vi "spectrometer-config.vi"(0 "Spectrograph Input Cluster":T3={"Slit Width (µm)"=50.0, "Diffraction Grating"=3, "Central Wavelength (nm)"=1000.0, "Filter"=4, "Shutter"=0} {"Shutter" items=["Close", "Open"]; "Slit Width (µm)" min=10.0 max=2500.0 step=0.1 format="%.1f"; "Diffraction Grating" items=["500 nm blaze"=1, "800 nm blaze"=2, "1250 nm blaze"=3]; "Filter" items=["Empty"=5, "Longpass 900 nm"=4, "Longpass 715 nm"=3, "Longpass 475 nm"=2, "Longpass 320 nm"=1]; "Central Wavelength (nm)" min=200.0 max=2000.0 step=0.1 format="%.1f"}, 2 "Initialization Successful?":bool, 3 "Spectrograph Reset Cluster":T1) -> (4 "Reset Control Cluster":T1, 5 "Spectrograph Output Cluster":T3={"Slit Width (µm)"=50.0, "Diffraction Grating"=3, "Central Wavelength (nm)"=1000.0, "Filter"=4, "Shutter"=0} {"Shutter" items=["Close", "Open"]; "Slit Width (µm)" min=10.0 max=2500.0 step=0.1 format="%.1f"; "Diffraction Grating" items=["500 nm blaze"=1, "800 nm blaze"=2, "1250 nm blaze"=3]; "Filter" items=["Empty"=5, "Longpass 900 nm"=4, "Longpass 715 nm"=3, "Longpass 475 nm"=2, "Longpass 320 nm"=1]; "Central Wavelength (nm)" min=200.0 max=2000.0 step=0.1 format="%.1f"}, 6 "Configuration Successful?":bool, 7 "Output Control Cluster":T2)   [LabVIEW 2015]
uses:
  <userlib>/Shamrock.llb/shamrock_autoSlit_typedef.ctl
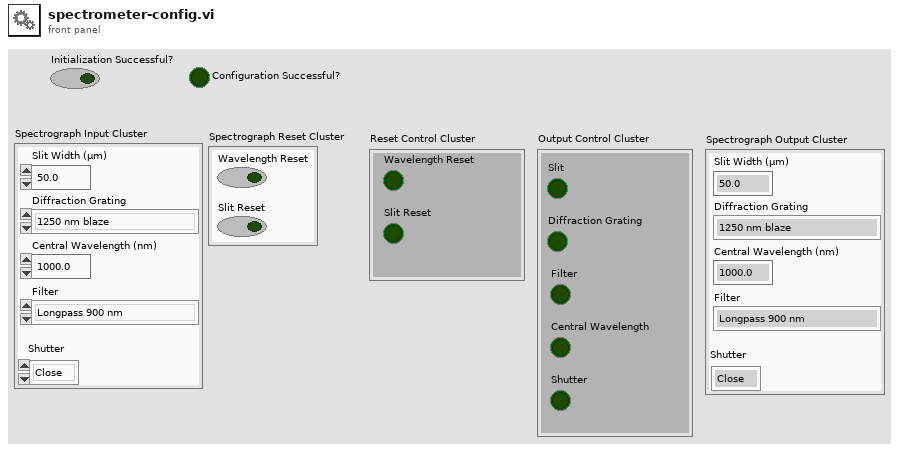
[diagram p1: front panel]
types:
  T1 = cluster{"Wavelength Reset":bool, "Slit Reset":bool}
  T2 = cluster{"Slit":bool, "Diffraction Grating":bool, "Filter":bool, "Central Wavelength":bool, "Shutter":bool}
  T3 = cluster{"Slit Width (µm)":dbl, "Diffraction Grating":u16, "Central Wavelength (nm)":dbl, "Filter":u16, "Shutter":u16}
  T4 = typedef "shamrock_autoSlit_typedef.ctl" = enum32{"Reserved (0)", "INPUT SIDE", "INPUT DIRECT", "OUTPUT SIDE", "OUTPUT DIRECT"}
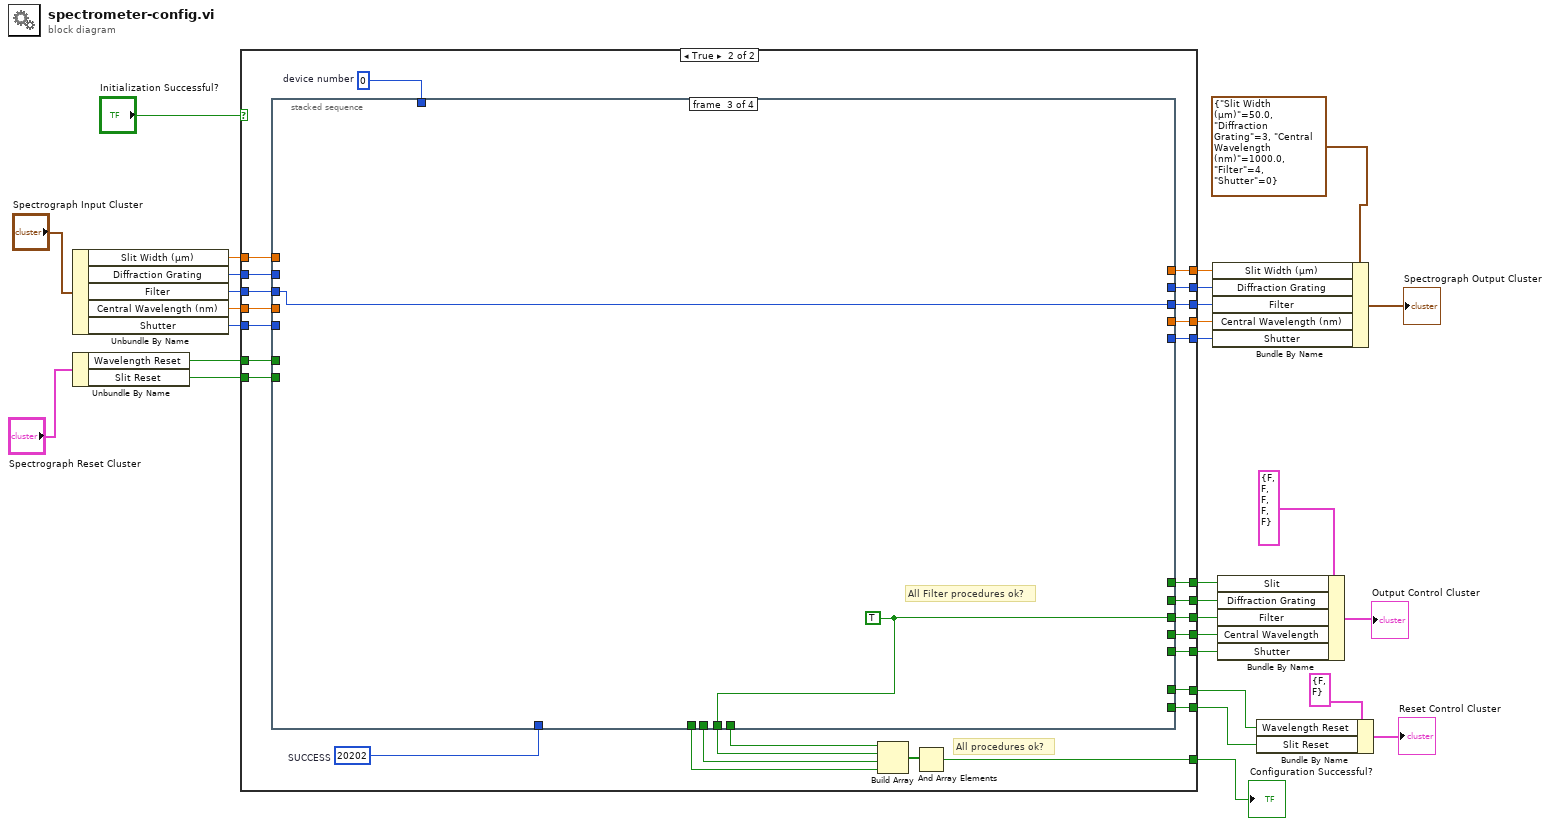
[diagram p0: block diagram]
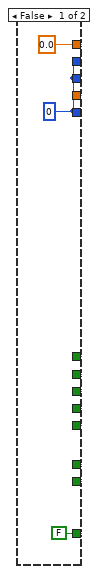
[diagram p2: hidden frame]
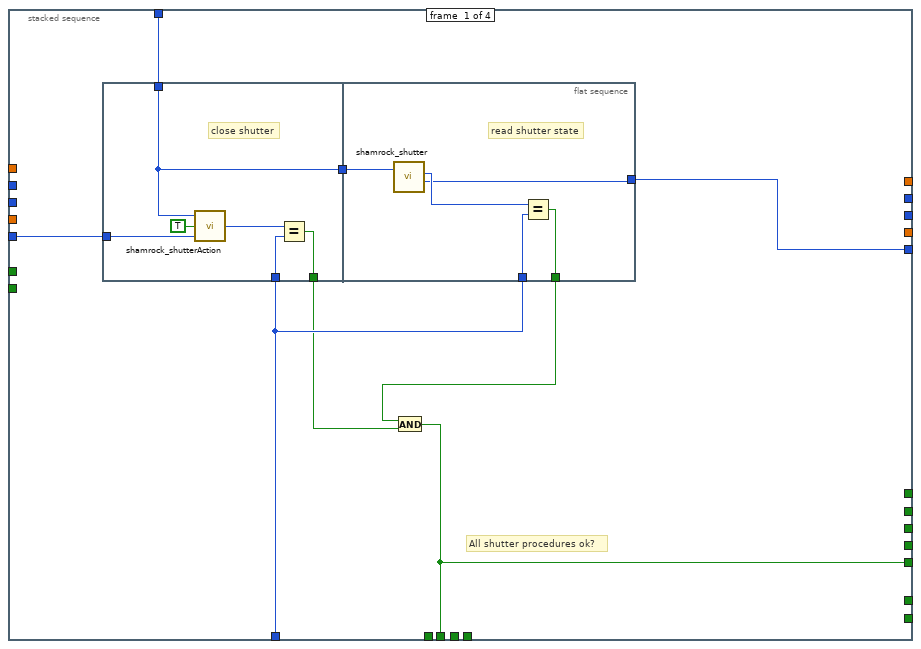
[diagram p3: hidden frame]
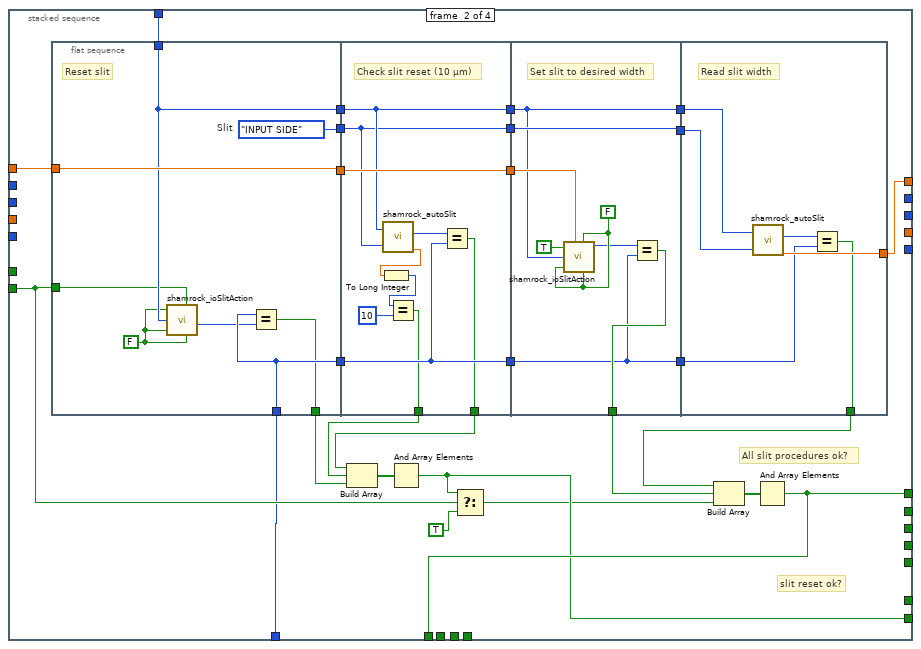
[diagram p4: hidden frame]
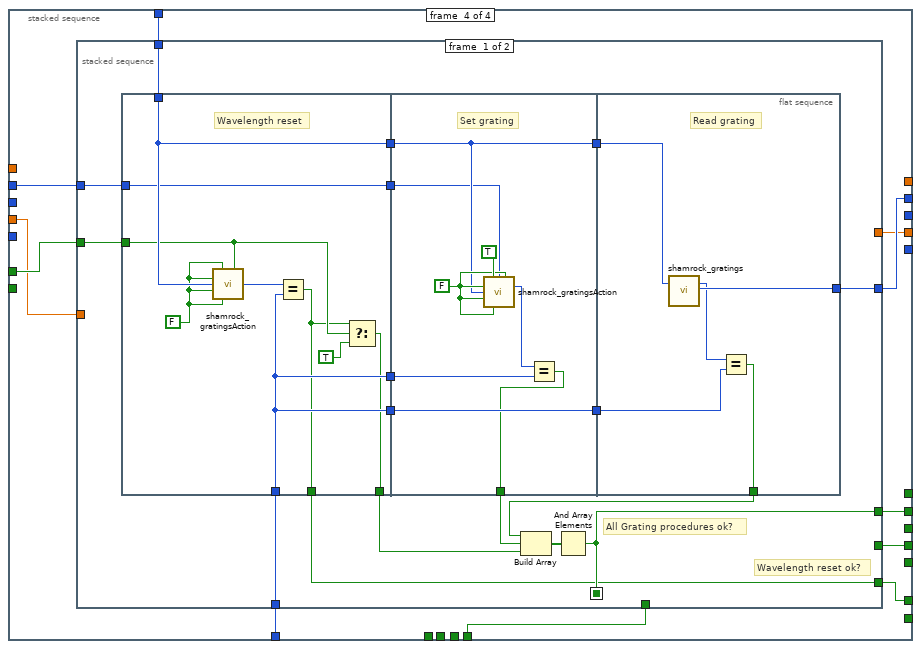
[diagram p5: hidden frame]
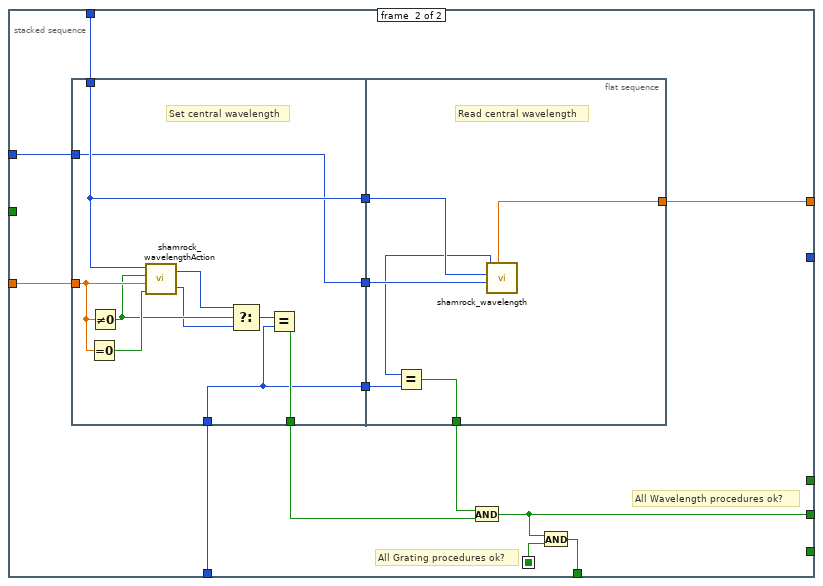
[diagram p6: hidden frame]
diagram:
  n1 = Unbundle By Name("Spectrograph Input Cluster") -> ("Slit Width (µm)"=w28:dbl, "Diffraction Grating"=w27:u16, "Filter"=w22:u16, "Central Wavelength (nm)"=w15:dbl, "Shutter"=w14:u16)
  n2 = Unbundle By Name("Spectrograph Reset Cluster") -> ("Wavelength Reset"=w24:bool, "Slit Reset"=w23:bool)
  n3 = case shown="True" "Initialization Successful?" {
    tunnel: [w30 w58] -> w29
    tunnel: w28 -> [_ w57]
    tunnel: w27 -> [_ w56]
    tunnel: w24 -> [_ w55]
    tunnel: w22 -> [_ w54]
    tunnel: w23 -> [_ w53]
    tunnel: w14 -> [_ w52]
    tunnel: w15 -> [_ w51]
    tunnel: [w32 w47] -> w20
    tunnel: [w31 w44] -> w19
    tunnel: [w30 w42] -> w4
    tunnel: [w30 w41] -> w6
    tunnel: [w30 w40] -> w5
    tunnel: [w30 w39] -> w8
    tunnel: [w32 w38] -> w17
    tunnel: [w30 w37] -> w7
    tunnel: [w31 w36] -> w18
    tunnel: [w31 w35] -> w16
    tunnel: [w30 w34] -> w11
    tunnel: [w30 w33] -> w10
    frame False {
      w31 = 0 ("Filter")
      w32 = 0.0 ("Slit width (mm)")
      w30 = FALSE
    }
    frame True {
      w49 = 20202  # SUCCESS
      w50 = 0  # device number
      # "All procedures ok?"
      n4 = stacked-sequence {
        tunnel: [w61 _ _ _] -> w59
        tunnel: w57 -> [_ w104 _ _]
        tunnel: w56 -> [_ _ _ w144]
        tunnel: w55 -> [_ _ _ w147]
        tunnel: w54 -> [_ _ w138 _]
        tunnel: w53 -> [_ w83 _ _]
        tunnel: w52 -> [w65 _ _ _]
        tunnel: w51 -> [_ _ _ w145]
        tunnel: w50 -> [w67 w105 _ w149]
        tunnel: w49 -> [w64 w79 _ w150]
        tunnel: [_ w89 _ _] -> w48
        tunnel: [_ w101 _ _] -> w47
        tunnel: [_ _ w139 _] -> w45
        tunnel: [_ _ _ w148] -> w44
        tunnel: [_ _ _ w142] -> w43
        tunnel: [w61 _ _ _] -> w42
        tunnel: [_ w89 _ _] -> w41
        tunnel: [_ _ w139 _] -> w40
        tunnel: [_ _ _ w146] -> w39
        tunnel: [_ _ _ w143] -> w38
        tunnel: [_ _ _ w141] -> w37
        tunnel: [_ _ w138 _] -> w36
        tunnel: [w60 _ _ _] -> w35
        tunnel: [_ w84 _ _] -> w34
        tunnel: [_ _ _ w140] -> w33
        frame #0 {
          # "All shutter procedures ok?"
          n5 = flat-sequence {
            tunnel: [w72] -> w62
            tunnel: w67 -> [w71]
            tunnel: [w71] -> w66
            tunnel: w65 -> [w68]
            tunnel: w64 -> [w69]
            tunnel: w66 -> [w78]
            tunnel: w64 -> [w77]
            tunnel: [w76] -> w63
            tunnel: [w74] -> w60
            frame #0 {
              # "close shutter"
              n6 = call <userlib>:"shamrock_shutterAction.vi"("Mode"=w68, "SetShutter"=TRUE, "Device No"=w71) -> ("SetShutter"=w70:u32)
              n7 = Equal?(x=w70, y=w69) -> (x = y?=w72:bool)
            }
            frame #1 {
              # "read shutter state"
              n8 = call <userlib>:"shamrock_shutter.vi"("Device No"=w78) -> ("GetShutter"=w75:u32, "Shutter"=w74:i32)  [unwired: 1 in, 4 out]
              n9 = Equal?(x=w75, y=w77) -> (x = y?=w76:bool)
            }
          }
          n10 = And(x=w63, y=w62) -> (x .and. y?=w61:bool)
        }
        frame #1 {
          # "slit reset ok?"
          # "All slit procedures ok?"
          n11 = flat-sequence {
            tunnel: w105 -> [w110]
            tunnel: w83 -> [w107]
            tunnel: w79 -> [w111]
            tunnel: w104 -> [w113]
            tunnel: [w113] -> w98
            tunnel: [w112] -> w96
            tunnel: [w110] -> w94
            tunnel: [w111] -> w92
            tunnel: [w106] -> w87
            tunnel: w98 -> [w123]
            tunnel: [w123] -> w97
            tunnel: w96 -> [w121]
            tunnel: [w121] -> w95
            tunnel: w94 -> [w122]
            tunnel: [w122] -> w93
            tunnel: w92 -> [w119]
            tunnel: [w119] -> w91
            tunnel: [w115] -> w86
            tunnel: [w114] -> w85
            tunnel: [w131] -> w80
            tunnel: w97 -> [w129]
            tunnel: w95 -> [w130]
            tunnel: w93 -> [w128]
            tunnel: w91 -> [w124]
            tunnel: [w128] -> w103
            tunnel: [w130] -> w102
            tunnel: [w124] -> w100
            tunnel: w103 -> [w137]
            tunnel: w102 -> [w133]
            tunnel: [w136] -> w101
            tunnel: w100 -> [w135]
            tunnel: [w134] -> w81
            frame #0 {
              w108 = FALSE ("SetSlit")
              w112 = shamrock_autoSlit_typedef."INPUT SIDE"  # Slit
              # "Reset slit"
              n12 = call <userlib>:"shamrock_ioSlitAction.vi"("SetSlit"=w108, "Device No"=w110, "SetOuputSlit"=w108, "Reset Slit"=w107, "Reset Output Slit"=w108) -> ("ResetSlit"=w109:u32)  [unwired: 2 in, 3 out]
              n13 = Equal?(x=w111, y=w109) -> (x = y?=w106:bool)
            }
            frame #1 {
              # "Check slit reset (10 µm)"
              n14 = call <userlib>:"shamrock_autoSlit.vi"("Device No"=w122, "Slit"=w121) -> ("RC_GetSlit"=w120:u32, "Slit width (mm)"=w117:dbl)  [unwired: 2 out]
              n15 = To Long Integer(number=w117) -> (32bit integer=w118:i32)
              n16 = Equal?(x=w118, y=10) -> (x = y?=w115:bool)
              n17 = Equal?(x=w120, y=w119) -> (x = y?=w114:bool)
            }
            frame #2 {
              w126 = FALSE ("Reset Slit")
              # "Set slit to desired width"
              n18 = call <userlib>:"shamrock_ioSlitAction.vi"("SetSlit"=TRUE, "Slit Width"=w129, "Device No"=w128, "SetOuputSlit"=w126, "Reset Slit"=w126, "Reset Output Slit"=w126) -> ("SetSlit"=w125:u32)  [unwired: 1 in, 3 out]
              n19 = Equal?(x=w125, y=w124) -> (x = y?=w131:bool)
            }
            frame #3 {
              # "Read slit width"
              n20 = call <userlib>:"shamrock_autoSlit.vi"("Device No"=w137, "Slit"=w133) -> ("RC_GetSlit"=w132:u32, "Slit width (mm)"=w136:dbl)  [unwired: 2 out]
              n21 = Equal?(x=w132, y=w135) -> (x = y?=w134:bool)
            }
          }
          n22 = Build Array(w85, w86, w87) -> (w88:bool[])
          n23 = And Array Elements(Boolean array=w88) -> (logical AND=w84:bool)
          n24 = Select(t=w84, s=w83, f=TRUE) -> (s? t:f=w82:bool)
          n25 = Build Array(w81, w80, w82) -> (w99:bool[])
          n26 = And Array Elements(Boolean array=w99) -> (logical AND=w89:bool)
        }
        frame #2 {
          w139 = TRUE ("x .and. y?")
          # "All Filter procedures ok?"
        }
        frame #3 {
          n27 = stacked-sequence {
            seq-local: [w152 _] -> [_ w193]
            tunnel: w150 -> [w167 w190]
            tunnel: w149 -> [w165 w202]
            tunnel: [w162 _] -> w148
            tunnel: w147 -> [w156 _]
            tunnel: [w152 _] -> w146
            tunnel: w145 -> [_ w201]
            tunnel: w144 -> [w153 w198]
            tunnel: [_ w194] -> w143
            tunnel: [_ w192] -> w142
            tunnel: [_ w191] -> w141
            tunnel: [w151 _] -> w140
            frame #0 {
              # "Wavelength reset ok?"
              # "All Grating procedures ok?"
              n28 = flat-sequence {
                tunnel: w167 -> [w174]
                tunnel: [w174] -> w166
                tunnel: w165 -> [w175]
                tunnel: [w175] -> w164
                tunnel: [w174] -> w161
                tunnel: w156 -> [w172]
                tunnel: [w170] -> w155
                tunnel: [w169] -> w154
                tunnel: w153 -> [w169]
                tunnel: [w168] -> w151
                tunnel: w166 -> [w182]
                tunnel: w164 -> [w180]
                tunnel: [w180] -> w163
                tunnel: w161 -> [w179]
                tunnel: [w179] -> w160
                tunnel: [w178] -> w158
                tunnel: w154 -> [w177]
                tunnel: w163 -> [w189]
                tunnel: [w188] -> w162
                tunnel: w160 -> [w186]
                tunnel: [w185] -> w159
                frame #0 {
                  w173 = FALSE ("SetTurret")
                  # "Wavelength reset"
                  n29 = call <userlib>:"shamrock_gratingsAction.vi"("WavelengthReset"=w172, "SetGrating"=w173, "SetGratingOffset"=w173, "SetTurret"=w173, "Device No"=w175, "SetDetectorOffset"=w173) -> ("WavelengthReset"=w176:u32)  [unwired: 5 in, 4 out]
                  n30 = Equal?(x=w176, y=w174) -> (x = y?=w168:bool)
                  n31 = Select(t=w168, s=w172, f=TRUE) -> (s? t:f=w170:bool)
                }
                frame #1 {
                  w181 = FALSE ("SetTurret")
                  # "Set grating"
                  n32 = call <userlib>:"shamrock_gratingsAction.vi"("WavelengthReset"=w181, "Grating"=w177, "SetGrating"=TRUE, "SetGratingOffset"=w181, "SetTurret"=w181, "Device No"=w180, "SetDetectorOffset"=w181) -> ("SetGrating"=w183:u32)  [unwired: 4 in, 4 out]
                  n33 = Equal?(x=w183, y=w182) -> (x = y?=w178:bool)
                }
                frame #2 {
                  # "Read grating"
                  n34 = call <userlib>:"shamrock_gratings.vi"("Device No"=w189) -> ("GetGrating"=w187:u32, "Grating"=w188:i32)  [unwired: 2 in, 15 out]
                  n35 = Equal?(x=w187, y=w186) -> (x = y?=w185:bool)
                }
              }
              n36 = Build Array(w159, w158, w155) -> (w157:bool[])
              n37 = And Array Elements(Boolean array=w157) -> (logical AND=w152:bool)
            }
            frame #1 {
              # "All Grating procedures ok?"
              # "All Wavelength procedures ok?"
              n38 = flat-sequence {
                tunnel: w202 -> [w212]
                tunnel: w201 -> [w207]
                tunnel: [w212] -> w200
                tunnel: [w211] -> w199
                tunnel: w198 -> [w211]
                tunnel: [w209] -> w197
                tunnel: [w210] -> w196
                tunnel: w190 -> [w209]
                tunnel: w200 -> [w218]
                tunnel: w199 -> [w217]
                tunnel: w197 -> [w215]
                tunnel: [w214] -> w195
                tunnel: [w213] -> w194
                frame #0 {
                  # "Set central wavelength"
                  n39 = Equal To 0?(x=w207) -> (x = 0?=w208:bool)
                  n40 = Not Equal To 0?(x=w207) -> (x != 0?=w206:bool)
                  n41 = call <userlib>:"shamrock_wavelengthAction.vi"("GoToZeroOrder"=w208, "Wavelength"=w207, "SetWavelength"=w206, "Device No"=w212) -> ("GotoZeroOrder"=w204:u32, "SetWavelength"=w205:u32)
                  n42 = Select(t=w205, s=w206, f=w204) -> (s? t:f=w203:u32)
                  n43 = Equal?(x=w203, y=w209) -> (x = y?=w210:bool)
                }
                frame #1 {
                  # "Read central wavelength"
                  n44 = call <userlib>:"shamrock_wavelength.vi"("Grating No"=w217, "Device No"=w218) -> ("GetWavelength"=w216:u32, "Wavelength"=w213:dbl)  [unwired: 7 out]
                  n45 = Equal?(x=w216, y=w215) -> (x = y?=w214:bool)
                }
              }
              n46 = And(x=w195, y=w196) -> (x .and. y?=w191:bool)
              n47 = And(x=w191, y=w193) -> (x .and. y?=w192:bool)
            }
          }
        }
      }
      n48 = Build Array(w43, w45, w59, w48) -> (w46:bool[])
      n49 = And Array Elements(Boolean array=w46) -> (logical AND=w58:bool)
    }
  }
  "Configuration Successful?" <- w29
  n50 = Bundle By Name(cluster=T3 {"Slit Width (µm)"=50.0, "Diffraction Grating"=3, "Central Wavelength (nm)"=1000.0, "Filter"=4, "Shutter"=0} ("Spectrograph Output Cluster"), "Slit Width (µm)"=w20, "Diffraction Grating"=w19, "Filter"=w18, "Central Wavelength (nm)"=w17, "Shutter"=w16) -> (→"Spectrograph Output Cluster":T3)
  n51 = Bundle By Name(cluster=T2 {"Slit"=FALSE, "Diffraction Grating"=FALSE, "Filter"=FALSE, "Central Wavelength"=FALSE, "Shutter"=FALSE} ("Output Control Cluster"), "Slit"=w6, "Diffraction Grating"=w8, "Filter"=w5, "Central Wavelength"=w7, "Shutter"=w4) -> (→"Output Control Cluster":T2)
  n52 = Bundle By Name(cluster=T1 {"Wavelength Reset"=FALSE, "Slit Reset"=FALSE} ("Reset Control Cluster"), "Wavelength Reset"=w10, "Slit Reset"=w11) -> (→"Reset Control Cluster":T1)
